vi "Example Simple.vi"() -> ()   [LabVIEW 2010]
uses:
  C:/tf/play/labview/Tinkerforge.dll
panel:
  in  "uid":string="amb"
  in  "port":i32=4223
  in  "host":string="localhost"
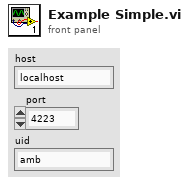
[diagram p1: front panel]
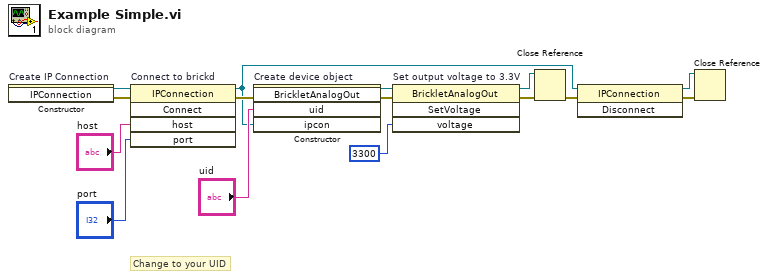
[diagram p0: block diagram]
diagram:
  # "Change to your UID"
  n1 = constructor on="Create IP Connection" class="IPConnection"() -> (reference out=w15:refnum<k24>, error out=w1:errorcluster)  [unwired: 3 in, 1 out]
  n2 = invoke on="Connect to brickd" class="IPConnection" method="Connect"(reference=w15, error in=w1, "host"="host", "port"="port") -> (reference out=w4:refnum<k24>, error out=w11:errorcluster)  [unwired: 1 in, 3 out]
  n3 = constructor on="Create device object" class="BrickletAnalogOut"(error in=w11, "uid"="uid", "ipcon"=w4) -> (reference out=w9:refnum<k24>, error out=w10:errorcluster)  [unwired: 2 in, 3 out]
  n4 = invoke on="Set output voltage to 3.3V" class="BrickletAnalogOut" method="SetVoltage"(reference=w9, error in=w10, "voltage"=3300) -> (reference out=w7:refnum<k24>, error out=w8:errorcluster)  [unwired: 1 in, 2 out]
  n5 = Close Reference(reference=w7, error in (no error)=w8) -> (error out=w6:errorcluster)
  n6 = invoke class="IPConnection" method="Disconnect"(reference=w4, error in=w6) -> (reference out=w3:refnum<k24>, error out=w5:errorcluster)  [unwired: 1 in, 1 out]
  n7 = Close Reference(reference=w3, error in (no error)=w5) -> ()  [unwired: 1 out]
